vi "Periodic Tasks.vi"(8 "error in":errorcluster) -> ()   [LabVIEW 2014]
doc: "This VI runs in parallel to other tasks. It can contain as many user-defined periodic loops as you need. These can carry out PID or other sorts of timed response."
uses:
  <vilib>/Rock Robotics/WPI/Relay/WPI_RelayValue.ctl
  <vilib>/Rock Robotics/SystemInterfaces/Utilities/FPGA_UtilitiesLED Source.ctl
  <vilib>/Rock Robotics/SystemInterfaces/Utilities/FPGA_UtilitiesLED State.ctl
  Robot Global Data.vi
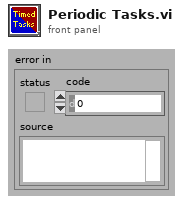
[diagram p1: front panel]
types:
  T1 = typedef "WPI_RelayValue.ctl" = enum16{"Off", "On", "Forward", "Reverse"}
  T2 = typedef "FPGA_UtilitiesLED State.ctl" = enum16{"Off", "On", "Toggle"}
  T3 = typedef "FPGA_UtilitiesLED Source.ctl" = enum16{"User LED", "FPGA LED"}
  T4 = typedef "WPI_CameraDevRef.ctl" = cluster{"Camera Address":string, "CameraStatus":errorcluster}
  T5 = typedef "WPI_MotorControlDeviceRef.ctl" = cluster{"DeviceStatus":errorcluster, "Type":T6, "PWM":cluster{"Controller":T7, "PWM Channel":T8, "DeadBand":T9}, "CAN":cluster{"Device Number":u8, "Control Mode":T10, "Semaphore":T11, "Max Vout":dbl, "TalonSRX Control Mode":T12}, "Invert":bool, "TransformRef":T13, "InvTransformRef":T13}
  T6 = typedef "WPI_MotorControlType.ctl" = enum16{"PWM", "CAN", "CANTalonSRX"}
  T7 = typedef "FPGA_TypedefDigitalModule.ctl" = enum16{"Controller 1"}
  T8 = typedef "FPGA_DIOPWMChannel.ctl" = enum8{"PWM 0", "PWM 1", "PWM 2", "PWM 3", "PWM 4", "PWM 5", "PWM 6", "PWM 7", "PWM 8", "PWM 9", "PWM MXP 0", "PWM MXP 1", "PWM MXP 2", "PWM MXP 3", "PWM MXP 4", "PWM MXP 5", "PWM MXP 6", "PWM MXP 7", "PWM MXP 8", "PWM MXP 9", "Invalid"}
  T9 = typedef "WPI_PWMDeadband.ctl" = cluster{"Name":string, "maxPositivePwm":i32, "minPositivePwm":i32, "centerPwm":i32, "maxNegativePwm":i32, "minNegativePwm":i32, "angularRange":u16}
  T10 = typedef "WPI_CANJaguar_ControlMode.ctl" = enum8{"Percent VBus", "Current", "Speed", "Position", "Voltage"}
  T11 = typedef "Semaphore RefNum" = refnum<k1>
  T12 = typedef "WPI_CANTalonSRX_APIControlMode.ctl" = enum8{"Percent VBus", "Speed", "Position", "Slave", "Unchanged / Invalid"}
  T13 = typedef "WPI_PWMTransform_ConPane.ctl" = refnum<vi>
  T14 = typedef "WPI_RelayDevRef.ctl" = cluster{"DevStatus":errorcluster, "Relay Channel":T15, "Controller":T7, "Relay Direction":T16}
  T15 = typedef "FPGA_DIORelayChannel.ctl" = enum8{"Relay 0", "Relay 1", "Relay 2", "Relay 3", "Invalid"}
  T16 = typedef "WPI_RelayDirection.ctl" = enum16{"Both directions", "Forward only", "Reverse only"}
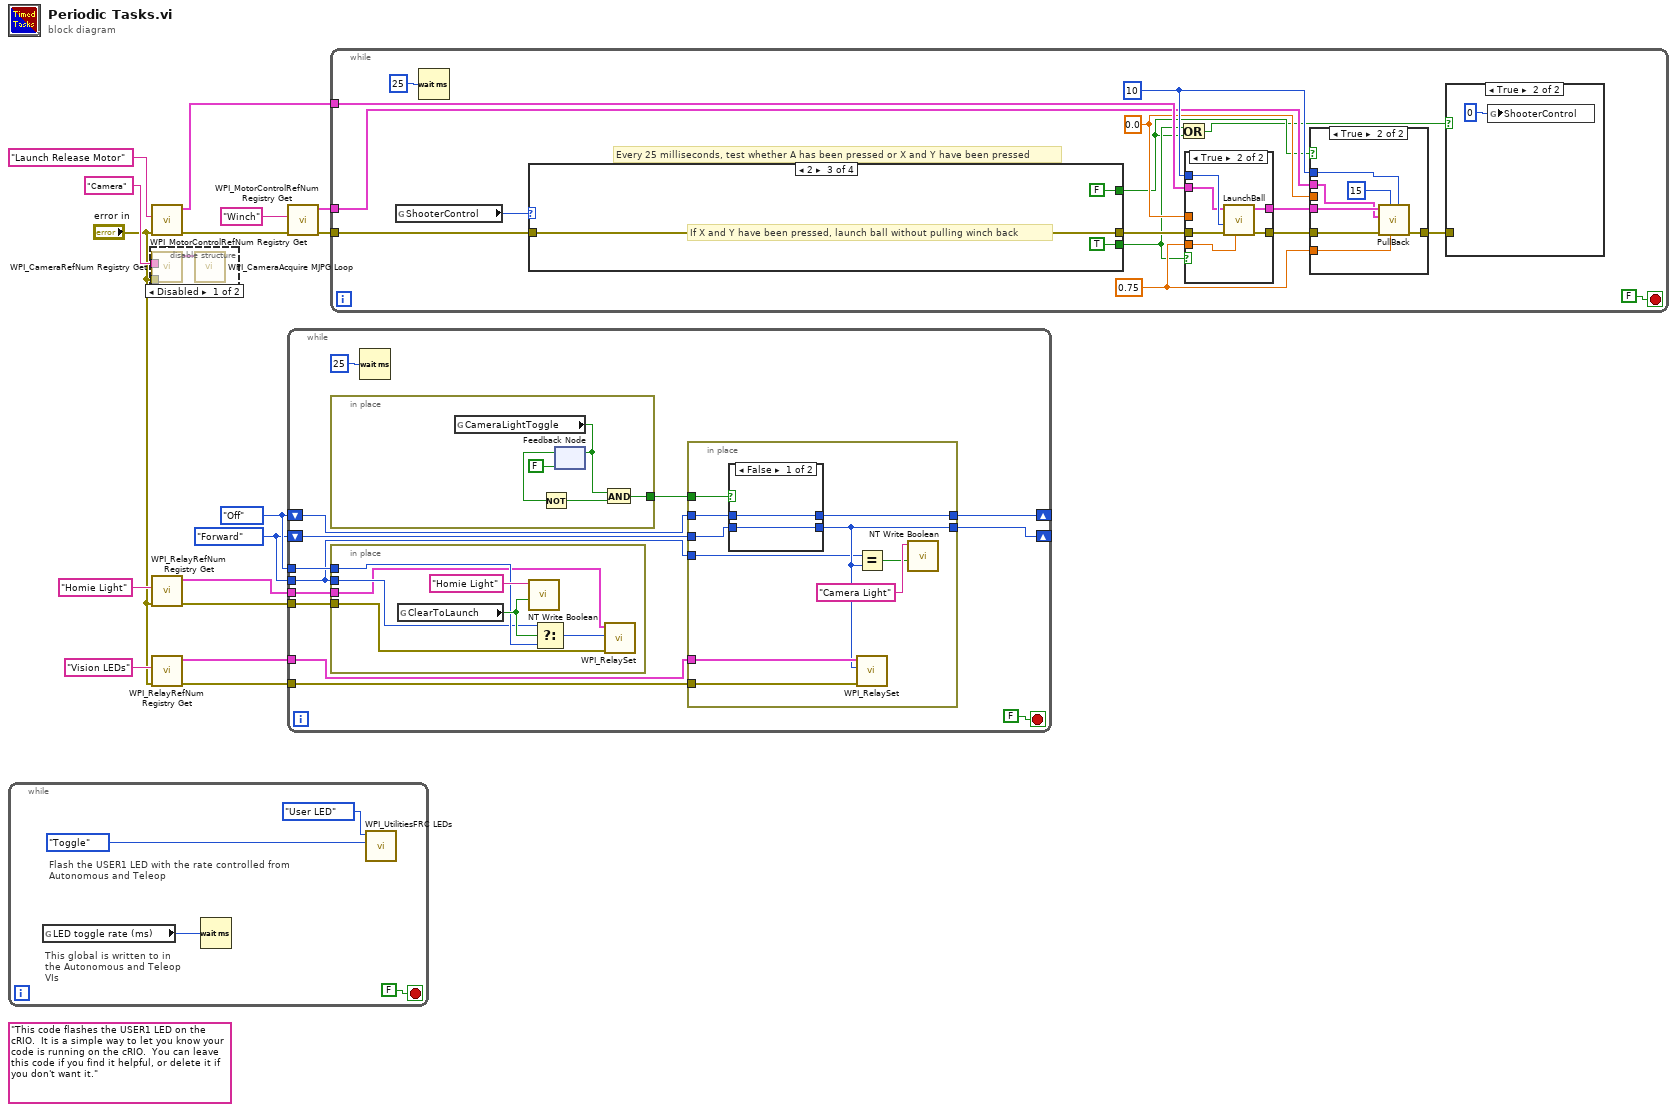
[diagram p0: block diagram]
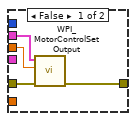
[diagram p5: hidden frame]
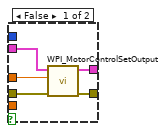
[diagram p6: hidden frame]
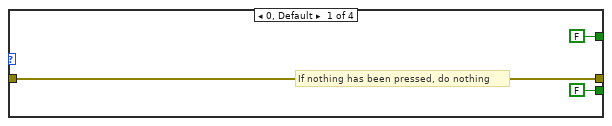
[diagram p7: hidden frame]
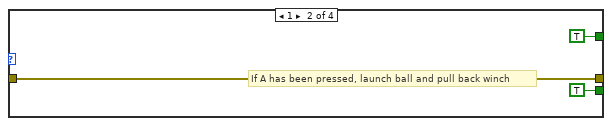
[diagram p8: hidden frame]
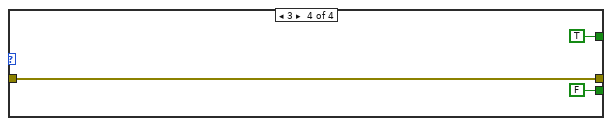
[diagram p9: hidden frame]
diagram:
  w3 = WPI_RelayValue."Off" ("t")
  w2 = WPI_RelayValue."Forward" ("RelayValue")
  (unwired) "This code flashes the USER1 LED on the cRIO.  It is a simple way to let you know your code is running on the cRIO.  You can leave this code if you find it helpful, or delete it if you don't want it."
  n1 = while {
    stop <- FALSE stop-if-true
    # "This global is written to in the Autonomous and Teleop VIs"
    # "Flash the USER1 LED with the rate controlled from Autonomous and Teleop"
    n2 = global read "Robot Global Data.vi" "LED toggle rate (ms)"() -> (w17:u32)
    n3 = Wait (ms)(milliseconds to wait=w17) -> ()  [unwired: 1 out]
    n4 = call <vilib>:"WPI_UtilitiesFRC LEDs.vi"("State"=FPGA_UtilitiesLED_State."Toggle", "LED Type"=FPGA_UtilitiesLED_Source."User LED") -> ()  [unwired: 1 in, 9 out]
  }
  n5 = disable-structure shown="Disabled" {
    disable-tunnel: "Camera" ("refnum name") -> [w23 _]
    disable-tunnel: "error in" -> [w21 _]
    frame Disabled {
      n6 = call <vilib>:"WPI_CameraRefNum Registry Get.vi"("error in (no error)"=w21, "refnum name"=w23) -> ("CameraDevRef"=w22:T4)  [unwired: 8 in, 1 out]
      n7 = call <vilib>:"WPI_CameraAcquire MJPG Loop.vi"("CameraDevRef"=w22) -> ()  [unwired: 11 in]
    }
    frame Enabled {
    }
  }
  n8 = call <vilib>:"WPI_MotorControlRefNum Registry Get.vi"("error in (no error)"="error in", "refnum name"="Launch Release Motor") -> ("error out"=w13:errorcluster, "MotorControlDevRef"=w9:T5)  [unwired: 8 in]
  n9 = call <vilib>:"WPI_RelayRefNum Registry Get.vi"("error in (no error)"="error in", "refnum name"="Homie Light") -> ("error out"=w6:errorcluster, "RelayDevRef"=w4:T14)  [unwired: 8 in]
  n10 = call <vilib>:"WPI_RelayRefNum Registry Get.vi"("error in (no error)"="error in", "refnum name"="Vision LEDs") -> ("error out"=w5:errorcluster, "RelayDevRef"=w14:T14)  [unwired: 8 in]
  n11 = call <vilib>:"WPI_MotorControlRefNum Registry Get.vi"("error in (no error)"=w13, "refnum name"="Winch") -> ("error out"=w12:errorcluster, "MotorControlDevRef"=w8:T5)  [unwired: 8 in]
  n12 = while {
    tunnel: w14 -> [w31]
    tunnel: w3 -> [w34]
    tunnel: w2 -> [w24]
    tunnel: w6 -> [w33]
    shift-right: [w28] -> _
    shift-left: w2 -> [w26]
    shift-right: [w29] -> _
    shift-left: w3 -> [w25]
    tunnel: w5 -> [w30]
    tunnel: w4 -> [w27]
    stop <- FALSE stop-if-true
    n13 = in-place {
      in-place-border: [w51] -> w32
      n14 = global read "Robot Global Data.vi" "CameraLightToggle"() -> (w52:bool)
      n15 = feedback #1(FALSE ("CameraLightToggle")) -> (w53:bool)
      n16 = Not(x=w53) -> (.not. x?=w54:bool)
      n17 = feedback-in #1(w52) -> ()
      n18 = And(x=w52, y=w54) -> (x .and. y?=w51:bool)
    }
    n19 = in-place {
      in-place-border: w34 -> [w59]
      in-place-border: w24 -> [w58]
      in-place-border: w33 -> [w57]
      in-place-border: w27 -> [w56]
      n20 = global read "Robot Global Data.vi" "ClearToLaunch"() -> (w61:bool)
      n21 = call <vilib>:"NT Write Boolean.vi"("Boolean"=w61, "Name"="Homie Light") -> ()  [unwired: 9 in, 1 out]
      n22 = Select(t=w58, s=w61, f=w59) -> (s? t:f=w62:T1)
      n23 = call <vilib>:"WPI_RelaySet.vi"("error in (no error)"=w57, "RelayValue"=w62, "RelayDevRef"=w56) -> ()  [unwired: 7 in, 2 out]
    }
    n24 = Wait (ms)(milliseconds to wait=u32 25) -> ()  [unwired: 1 out]
    n25 = in-place {
      in-place-border: w30 -> [w46]
      in-place-border: w31 -> [w45]
      in-place-border: w26 -> [w44]
      in-place-border: w25 -> [w43]
      in-place-border: w32 -> [w41]
      in-place-border: [w42] -> w29
      in-place-border: [w38] -> w28
      in-place-border: w24 -> [w37]
      n26 = case shown="False" w41 {
        tunnel: w44 -> [w48 w50]
        tunnel: w43 -> [w47 w49]
        tunnel: [w47 w50] -> w42
        tunnel: [w48 w49] -> w38
        frame False {
        }
        frame True {
        }
      }
      n27 = Equal?(x=w37, y=w38) -> (x = y?=w39:bool)
      n28 = call <vilib>:"WPI_RelaySet.vi"("error in (no error)"=w46, "RelayValue"=w38, "RelayDevRef"=w45) -> ()  [unwired: 7 in, 2 out]
      n29 = call <vilib>:"NT Write Boolean.vi"("Boolean"=w39, "Name"="Camera Light") -> ()  [unwired: 9 in, 1 out]
    }
  }
  n30 = while {
    tunnel: w12 -> [w76]
    tunnel: w9 -> [w70]
    tunnel: w8 -> [w69]
    stop <- FALSE stop-if-true
    w68 = 0.0 ("Output")
    w71 = 0.75 ("Output")
    w73 = 10
    # "Every 25 milliseconds, test whether A has been pressed or X and Y have been pressed"
    n31 = global read "Robot Global Data.vi" "ShooterControl"() -> (w72:u32)
    n32 = Wait (ms)(milliseconds to wait=u32 25) -> ()  [unwired: 1 out]
    n33 = case shown="2" w72 {
      tunnel: w76 -> [w102 w105 w108 w111]
      tunnel: [w102 w105 w108 w111] -> w74
      tunnel: [FALSE TRUE TRUE FALSE] -> w65
      tunnel: [FALSE TRUE FALSE TRUE] -> w64
      frame 0, Default {
        # "If nothing has been pressed, do nothing"
      }
      frame 1 {
        # "If A has been pressed, launch ball and pull back winch"
      }
      frame 2 {
        # "If X and Y have been pressed, launch ball without pulling winch back"
      }
      frame 3 {
      }
    }
    n34 = Or(x=w65, y=w64) -> (x .or. y?=w63:bool)
    n35 = case shown="True" w65 {
      tunnel: w74 -> [w93 w101]
      tunnel: [w95 w100] -> w75
      tunnel: w73 -> [_ w99]
      tunnel: w71 -> [_ w98]
      tunnel: w70 -> [w94 w97]
      tunnel: [w91 w96] -> w67
      tunnel: w68 -> [w92 _]
      frame False {
        n36 = call <vilib>:"WPI_MotorControlSetOutput.vi"("error in (no error)"=w93, "Output"=w92, "MotorControlDevRef"=w94) -> ("error out"=w95:errorcluster, "MotorControlDevRef"=w91:T5)  [unwired: 6 in, 1 out]
      }
      frame True {
        n37 = call "LaunchBall.vi"("Output"=w98, "error in (no error)"=w101, "Timeout (s)"=w99, "MotorControlDevRef"=w97) -> ("error out"=w100:errorcluster, "MotorControlDevRef 2"=w96:T5)  [unwired: 6 in]
      }
    }
    n38 = case shown="True" w64 {
      tunnel: w75 -> [w82 w89]
      tunnel: [w81 w90] -> w66
      tunnel: w73 -> [_ w86]
      tunnel: w71 -> [_ w88]
      tunnel: w67 -> [_ w85]
      tunnel: w69 -> [w80 w84]
      tunnel: w68 -> [w83 _]
      frame False {
        n39 = call <vilib>:"WPI_MotorControlSetOutput.vi"("error in (no error)"=w82, "Output"=w83, "MotorControlDevRef"=w80) -> ("error out"=w81:errorcluster)  [unwired: 6 in, 2 out]
      }
      frame True {
        n40 = call "PullBack.vi"("dog shifter timeout (s)"=w86, "Output"=w88, "winch timeout (s)"=15 ("Timeout (s)"), "error in (no error)"=w89, "WinchControlDevRef"=w84, "LaunchReleaseMotorControlDevRef"=w85) -> ("error out"=w90:errorcluster)  [unwired: 3 in, 2 out]
      }
    }
    n41 = case shown="True" w63 {
      tunnel: w66 -> [_ _]
      frame False {
      }
      frame True {
        n42 = global write "Robot Global Data.vi" "ShooterControl"(u32 0 ("ShooterControl")) -> ()
      }
    }
  }
